vi "Bus Interface.vi"(0 "stream control":refnum<class "niUSRP Stream Control (DMA) v1 FPGA.lvclass">, 1 "abort":bool, 5 "instruction":T2, 9 "input valid":bool) -> (6 "response":T1, 10 "done":bool, 14 "ready for input":bool)   [LabVIEW 2025, in "niUSRP Stream Control (DMA) v1 FPGA.lvclass"]
uses:
  niUSRP Stream Control (DMA) v1 FPGA.lvclass
  <instrlib>/_niInstr/Instruction Framework/v1/FPGA/Interfaces/Address Space/Address Space Instruction.ctl
  <instrlib>/_niInstr/Instruction Framework/v1/FPGA/Typedefs/Response.ctl
  niUSRP Stream Control (DMA) v1 FPGA.lvclass/niUSRP Stream Control (DMA) v1 FPGA.ctl
  <vilib>/rvi/DataTransferAndStorage/Container/Common/niFpgaContainerExecOnDevCompGetState.vi
  <vilib>/rvi/Emulation/niFpgaEmulationIsFPGAContextNoSignature.vi
  <vilib>/rvi/DataTransferAndStorage/Container/Common/niFpgaContainerGetUniqueNameForEmu.vi
  <vilib>/rvi/Memory/Memory_Emulation/niFpgaMemoryEmulationCacheClearOnFirstRun.vi
  <vilib>/rvi/Memory/Memory_Emulation/nirvimemoryEmulationManagerCache_MakeExclusive.vi
  <vilib>/rvi/Memory/Memory_Emulation/niFpgaMemoryEmulationValidateCache.vi
  <vilib>/rvi/Memory/Memory_Emulation/nirvimemoryEmulationManagerCache_InsertValue.vi
  <vilib>/Utility/error.llb/Clear Errors.vi
  <vilib>/rvi/Memory/Memory_Emulation/nirvimemoryEmulationManagerCache_ReleaseExclusive.vi
  <vilib>/rvi/Memory/Memory_Emulation/nirvimemoryEmulationManagerCache_GetValue.vi
  <vilib>/rvi/Memory/Memory_Emulation/nirvimemoryEmulationManagerCache_SetValue.vi
  <vilib>/rvi/Emulation/niFpgaProcessEmulError.vi
  <vilib>/rvi/Emulation/niFpgaSctlEmulationGetInTimedLoop.vi
  <vilib>/rvi/DataTransferAndStorage/Container/XNode/niFpgaContainer.xnode
  <vilib>/rvi/DataTransferAndStorage/Register/Emulation/niFpgaRegisterEmulationRefIn.vi
  <instrlib>/_niInstr/Instruction Framework/v1/FPGA/Typedefs/niInstr Instruction Framework v1 FPGA.lvlib
  <instrlib>/_niInstr/Instruction Framework/v1/FPGA/Interfaces/Address Space/Address Space.lvclass
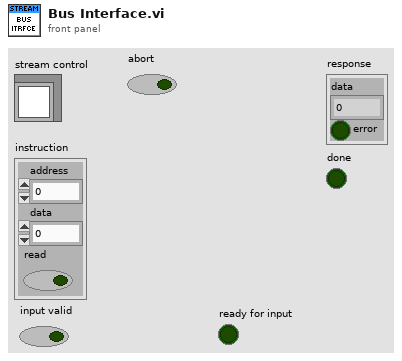
[diagram p1: front panel]
types:
  T1 = typedef "niInstr Instruction Framework v1 FPGA.lvlib/Response.ctl" = cluster{"data":u64, "error":bool}
  T2 = typedef "niInstr Instruction Framework Interfaces v1 FPGA.lvlib/Address Space.lvclass/Address Space Instruction.ctl" = cluster{"address":u32, "data":u64, "read":bool}
  T3 = typedef "niUSRP Stream Control (DMA) v1 FPGA.lvclass/Regs.ctl" = cluster{"stream enable":refnum<k21>, "reset":refnum<k21>, "abort":refnum<k21>, "start":refnum<k21>, "state":refnum<k21>, "samples processed (U32)":refnum<k21>, "under/overflows (U32)":refnum<k21>, "burst size (U32)":refnum<k21>, "rx fifo 0":refnum<k21>, "rx fifo 4spc":refnum<k21>, "tx fifo 0":refnum<k21>, "tx fifo 4spc":refnum<k21>, "enabled channels":refnum<k21>, "num channels":refnum<k21>, "SPC":u8, "end continuous mode":refnum<k21>, "stream start time":refnum<k21>}
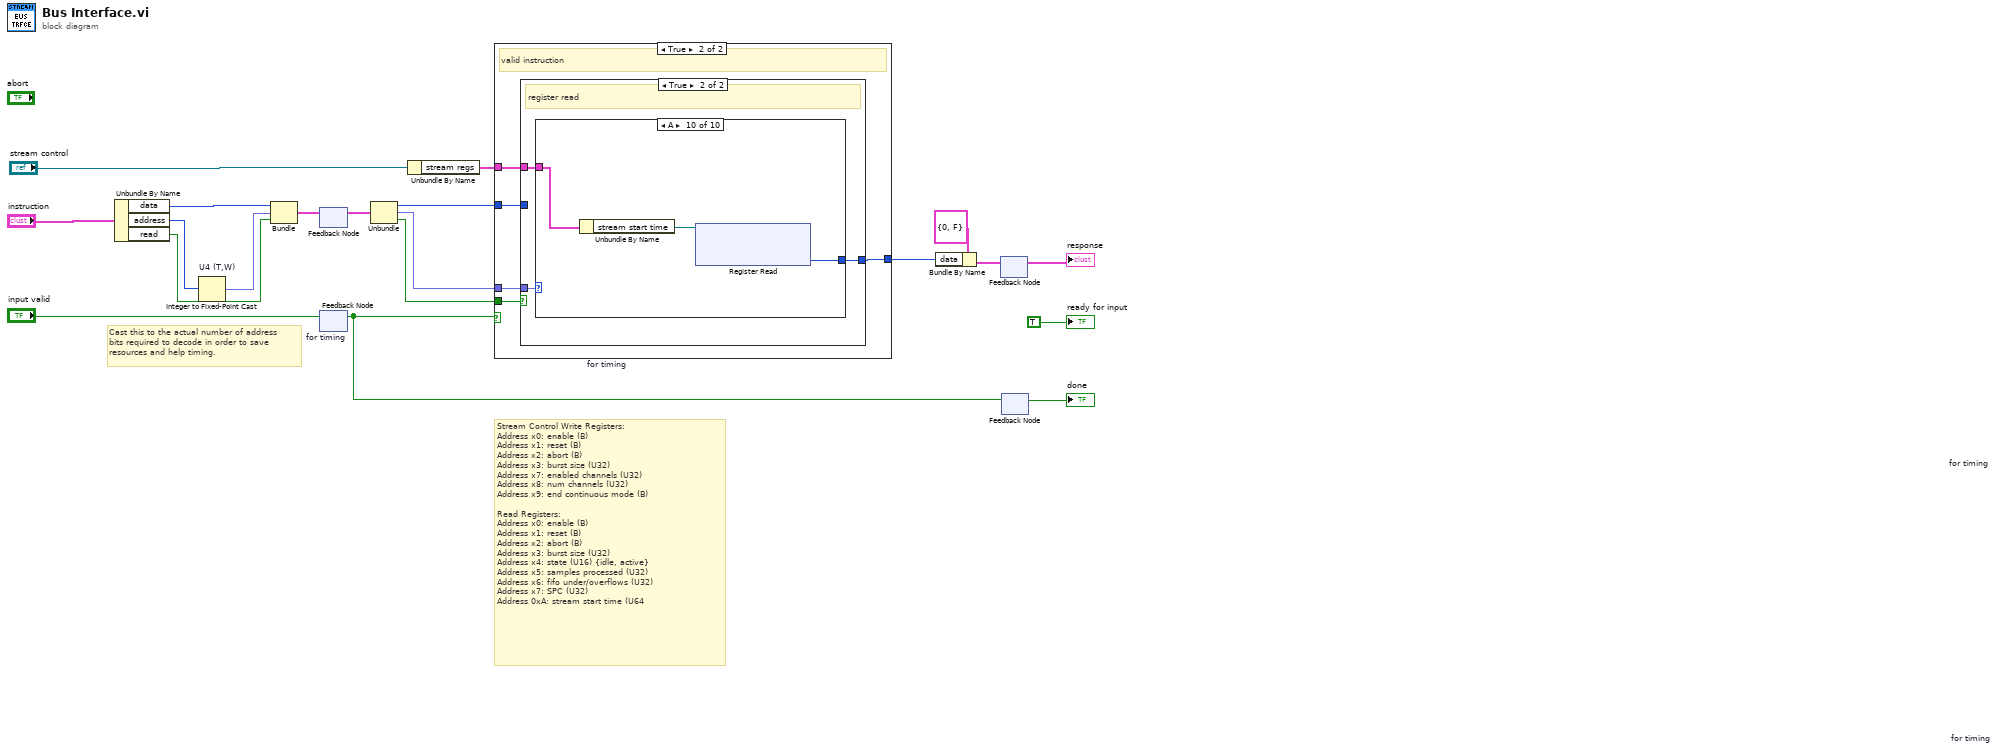
[diagram p0: block diagram]
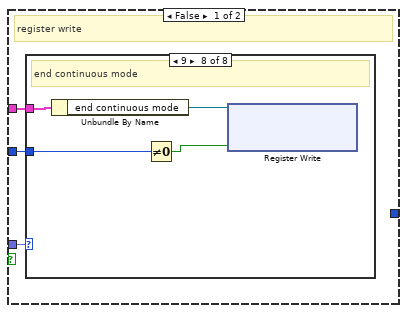
[diagram p3: hidden frame]
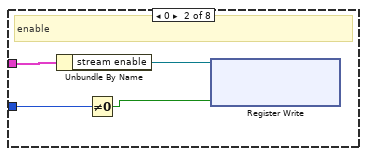
[diagram p5: hidden frame]
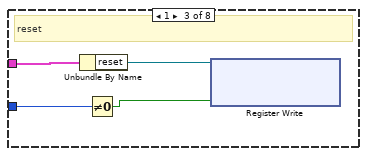
[diagram p6: hidden frame]
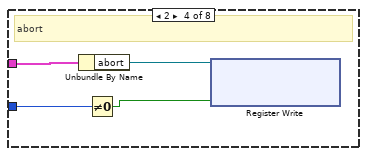
[diagram p7: hidden frame]
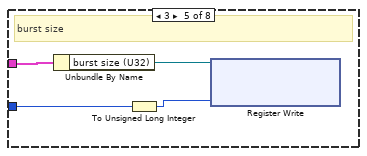
[diagram p8: hidden frame]
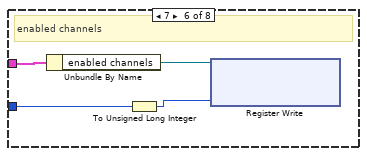
[diagram p9: hidden frame]
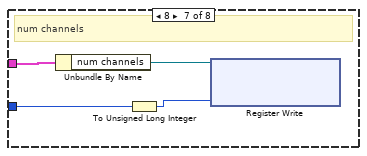
[diagram p10: hidden frame]
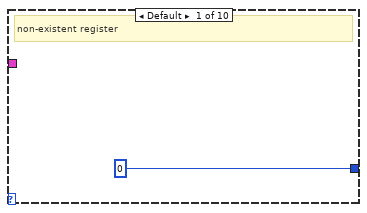
[diagram p11: hidden frame]
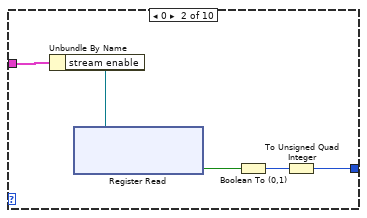
[diagram p12: hidden frame]
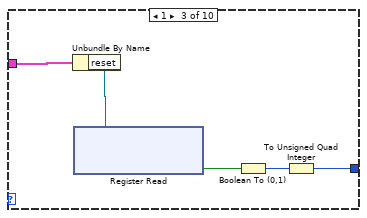
[diagram p13: hidden frame]
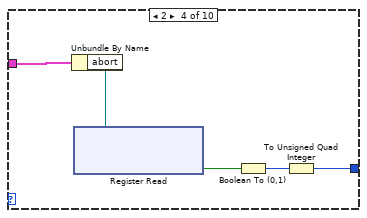
[diagram p14: hidden frame]
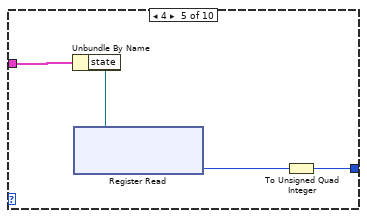
[diagram p15: hidden frame]
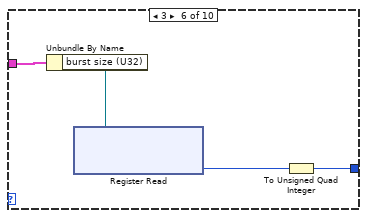
[diagram p16: hidden frame]
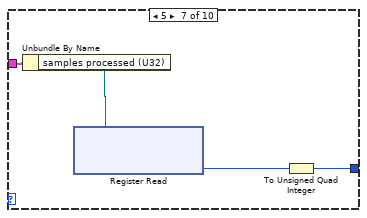
[diagram p17: hidden frame]
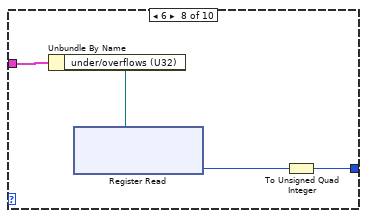
[diagram p18: hidden frame]
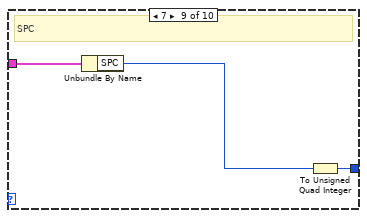
[diagram p19: hidden frame]
diagram:
  # "Stream Control Write Registers:\nAddress x0: enable (B)\nAddress x1: reset (B)\nAddress x2: abort (B)\nAddress x3: burst size (U32)\nAddress x7: enabled channels (U32)\nAddress x8: num channels (U32)\nAddress x9: end continuous mode (B)\n\nRead Registers:\nAddress x0: enable (B)\nAddress x1: reset (B)\nAddress x2: abort (B)\nAddress x3: burst size (U32)\nAddress x4: state (U16) {idle, active}\nAddress x5: samples processed (U32)\nAddress x6: fifo under/overflows (U32)\nAddress x7: SPC (U32)\nAddress 0xA: stream start time (U64"
  # "Cast this to the actual number of address\nbits required to decode in order to save\nresources and help timing."
  n1 = Unbundle By Name("instruction") -> ("data"=w17:u64, "address"=w20:u32, "read"=w15:bool)
  n2 = Integer to Fixed-Point Cast "U4 (T,W)"(integer=w20) -> (fixed-point=w16:fxp<+,4,4>)  [unwired: 1 in]
  n3 = Bundle("data"=w17, w16, "read"=w15) -> (w19:cluster{"data":u64, fxp<+,4,4>, "read":bool})  [unwired: 1 in]
  n4 = feedback #1 "for timing"() -> (w18:cluster{"data":u64, fxp<+,4,4>, "read":bool})  [unwired: 1 in]
  n5 = feedback-in #1(w19) -> ()
  n6 = feedback #2 "for timing"() -> (w1:bool)  [unwired: 1 in]
  n7 = feedback-in #2("input valid") -> ()
  n8 = Unbundle(w18) -> ("data"=w8:u64, w9:fxp<+,4,4>, "read"=w10:bool)
  n9 = Unbundle By Name("stream control") -> ("stream regs"=w11:T3)
  n10 = case shown="True" w1 {
    tunnel: w11 -> [_ w25]
    tunnel: w10 -> [_ w24]
    tunnel: w9 -> [_ w23]
    tunnel: w8 -> [_ w22]
    tunnel: [_ w21] -> w7
    frame False {
      # "invalid instruction"
    }
    frame True {
      # "valid instruction"
      n11 = case shown="True" w24 {
        tunnel: w23 -> [w28 w59]
        tunnel: [_ w58] -> w21
        tunnel: w22 -> [w27 _]
        tunnel: w25 -> [w26 w57]
        frame False {
          # "register write"
          n12 = case shown="9" w28 {
            tunnel: w27 -> [_ w30 w34 w38 w41 w45 w49 w54]
            tunnel: w26 -> [_ w31 w35 w39 w43 w47 w51 w53]
            frame Default {
              # "non-existent register"
            }
            frame 0 {
              # "enable"
              n13 = Unbundle By Name(w31) -> ("stream enable"=w32:refnum<k21>)
              n14 = Not Equal To 0?(x=w30) -> (x != 0?=w29:bool)
              n15 = xnode ("Register Write")("Data"=w29, "Register In"=w32) -> ()  [unwired: 1 out]
            }
            frame 1 {
              # "reset"
              n16 = Unbundle By Name(w35) -> ("reset"=w36:refnum<k21>)
              n17 = Not Equal To 0?(x=w34) -> (x != 0?=w33:bool)
              n18 = xnode ("Register Write")("Data"=w33, "Register In"=w36) -> ()  [unwired: 1 out]
            }
            frame 2 {
              # "abort"
              n19 = Unbundle By Name(w39) -> ("abort"=w40:refnum<k21>)
              n20 = Not Equal To 0?(x=w38) -> (x != 0?=w37:bool)
              n21 = xnode ("Register Write")("Data"=w37, "Register In"=w40) -> ()  [unwired: 1 out]
            }
            frame 3 {
              # "burst size"
              n22 = Unbundle By Name(w43) -> ("burst size (U32)"=w44:refnum<k21>)
              n23 = To Unsigned Long Integer(number=w41) -> (unsigned 32bit integer=w42:u32)
              n24 = xnode ("Register Write")("Data"=w42, "Register In"=w44) -> ()  [unwired: 1 out]
            }
            frame 7 {
              # "enabled channels"
              n25 = Unbundle By Name(w47) -> ("enabled channels"=w48:refnum<k21>)
              n26 = To Unsigned Long Integer(number=w45) -> (unsigned 32bit integer=w46:u32)
              n27 = xnode ("Register Write")("Data"=w46, "Register In"=w48) -> ()  [unwired: 1 out]
            }
            frame 8 {
              # "num channels"
              n28 = Unbundle By Name(w51) -> ("num channels"=w52:refnum<k21>)
              n29 = To Unsigned Long Integer(number=w49) -> (unsigned 32bit integer=w50:u32)
              n30 = xnode ("Register Write")("Data"=w50, "Register In"=w52) -> ()  [unwired: 1 out]
            }
            frame 9 {
              # "end continuous mode"
              n31 = Unbundle By Name(w53) -> ("end continuous mode"=w56:refnum<k21>)
              n32 = Not Equal To 0?(x=w54) -> (x != 0?=w55:bool)
              n33 = xnode ("Register Write")("Data"=w55, "Register In"=w56) -> ()  [unwired: 1 out]
            }
          }
        }
        frame True {
          # "register read"
          n34 = case shown="A" w59 {
            tunnel: [u64 0 w65 w70 w75 w79 w83 w87 w91 w94 w95] -> w58
            tunnel: w57 -> [_ w63 w68 w73 w77 w81 w85 w89 w93 w97]
            frame Default {
              # "non-existent register"
            }
            frame 0 {
              n35 = Unbundle By Name(w63) -> ("stream enable"=w64:refnum<k21>)
              n36 = xnode ("Register Read")("Register In"=w64) -> ("Data"=w62:bool)  [unwired: 1 out]
              n37 = Boolean To (0,1)(Boolean=w62) -> (0, 1=w61:i16)
              n38 = To Unsigned Quad Integer(1:w61) -> (0:w65:u64)
            }
            frame 1 {
              n39 = Unbundle By Name(w68) -> ("reset"=w69:refnum<k21>)
              n40 = xnode ("Register Read")("Register In"=w69) -> ("Data"=w67:bool)  [unwired: 1 out]
              n41 = Boolean To (0,1)(Boolean=w67) -> (0, 1=w66:i16)
              n42 = To Unsigned Quad Integer(1:w66) -> (0:w70:u64)
            }
            frame 2 {
              n43 = Unbundle By Name(w73) -> ("abort"=w74:refnum<k21>)
              n44 = xnode ("Register Read")("Register In"=w74) -> ("Data"=w72:bool)  [unwired: 1 out]
              n45 = Boolean To (0,1)(Boolean=w72) -> (0, 1=w71:i16)
              n46 = To Unsigned Quad Integer(1:w71) -> (0:w75:u64)
            }
            frame 4 {
              n47 = Unbundle By Name(w77) -> ("state"=w78:refnum<k21>)
              n48 = xnode ("Register Read")("Register In"=w78) -> ("Data"=w76:enum16{"Idle", "Active"})  [unwired: 1 out]
              n49 = To Unsigned Quad Integer(1:w76) -> (0:w79:u64)
            }
            frame 3 {
              n50 = Unbundle By Name(w81) -> ("burst size (U32)"=w82:refnum<k21>)
              n51 = xnode ("Register Read")("Register In"=w82) -> ("Data"=w80:u32)  [unwired: 1 out]
              n52 = To Unsigned Quad Integer(1:w80) -> (0:w83:u64)
            }
            frame 5 {
              n53 = Unbundle By Name(w85) -> ("samples processed (U32)"=w86:refnum<k21>)
              n54 = xnode ("Register Read")("Register In"=w86) -> ("Data"=w84:u32)  [unwired: 1 out]
              n55 = To Unsigned Quad Integer(1:w84) -> (0:w87:u64)
            }
            frame 6 {
              n56 = Unbundle By Name(w89) -> ("under/overflows (U32)"=w90:refnum<k21>)
              n57 = xnode ("Register Read")("Register In"=w90) -> ("Data"=w88:u32)  [unwired: 1 out]
              n58 = To Unsigned Quad Integer(1:w88) -> (0:w91:u64)
            }
            frame 7 {
              # "SPC"
              n59 = Unbundle By Name(w93) -> ("SPC"=w92:u8)
              n60 = To Unsigned Quad Integer(1:w92) -> (0:w94:u64)
            }
            frame 10 {
              n61 = Unbundle By Name(w97) -> ("stream start time"=w96:refnum<k21>)
              n62 = xnode "Register Read"("Register In"=w96) -> ("Data"=w95:u64)  [unwired: 1 out]
            }
          }
        }
      }
    }
  }
  n63 = Bundle By Name(cluster=T1 {"data"=0, "error"=FALSE} ("response"), "data"=w7) -> (w4:T1)
  n64 = feedback #3 "for timing"() -> (→"response":T1)  [unwired: 1 in]
  n65 = feedback-in #3(w4) -> ()
  n66 = feedback #4 "for timing"() -> (→"done":bool)  [unwired: 1 in]
  n67 = feedback-in #4(w1) -> ()
  "ready for input" <- TRUE ("ready for input")
